vi "Write DB.vi"(8 "error in (no error)":errorcluster, 10 "DB":refnum<class "Database.lvclass">, 11 "Form Model in":refnum<class "Form Model.lvclass">) -> (0 "error out":errorcluster, 3 "Form Model out":refnum<class "Form Model.lvclass">)   [LabVIEW 2020]
uses:
  Form Model.lvclass
  C:/Program Files (x86)/National Instruments/LabVIEW 2020/vi.lib/ActorFramework/Actor/Actor.lvclass
  C:/Users/User/Desktop/Raman Program/Database OOP/forms AF/Form Model/Form Model.lvclass
  source/Database/Database.lvclass
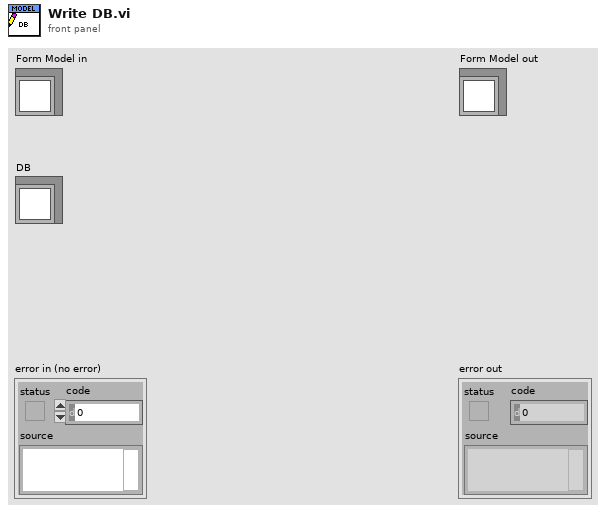
[diagram p1: front panel]
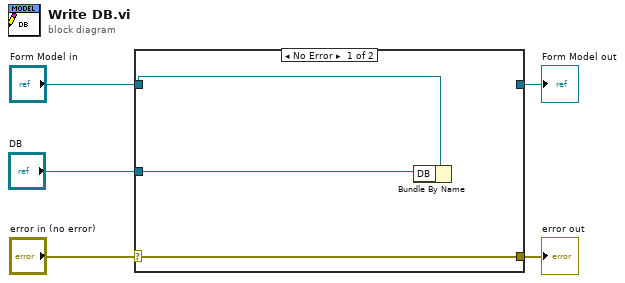
[diagram p0: block diagram]
diagram:
  n1 = case shown="No Error" "error in (no error)" {
    selector: "error in (no error)" -> [w8 w9]
    tunnel: [w8 w9] -> w4
    tunnel: [_ w10] -> w2
    tunnel: "Form Model in" -> [w6 w10]
    tunnel: "DB" -> [w7 _]
    frame No Error {
      n2 = Bundle By Name(cluster=w6, "DB"=w7) -> ()  [unwired: 1 out]
    }
    frame Error {
    }
  }
  "error out" <- w4
  "Form Model out" <- w2
